vi "Log Data.vi"(8 "error in (no error)":errorcluster, 11 "Historian Logger in":refnum<class "Historian Logger.lvclass">) -> (0 "error out":errorcluster, 3 "Historian Logger out":refnum<class "Historian Logger.lvclass">)   [LabVIEW 2020, in "VolatusHistorian.lvlib" / "Historian Logger.lvclass"]
uses:
  Historian Logger.lvclass
  Historian Logger.lvclass/Historian Logger.ctl
  lv-vecto/Vecto/Group DBL/Group DBL.lvclass
  Volatus/MessageQ/MessageQ.lvclass/MessageQ.ctl
  Volatus/MessageQ/Send.vi
  lv-vecto/Vecto/Group/Group.lvclass
  VolatusData/VolatusData.lvlib
  VolatusErrorUtilities/MultiErrors/MultiErrors.lvclass
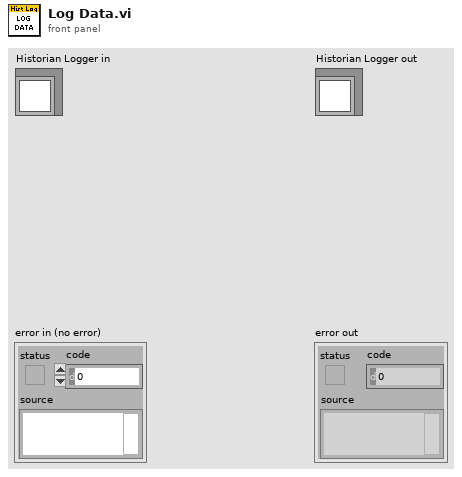
[diagram p1: front panel]
types:
  T1 = typedef "VolatusHistorian.lvlib/Historian Logger.lvclass/Group Info.ctl" = cluster{"Buffer":refnum<class "Group Buffer DBL.lvclass">, "Logger":refnum<class "MessageQ.lvclass">, "Group":refnum<class "Group.lvclass">, "Last Timestamp":dbl, "State":T2}
  T2 = typedef "VolatusData.lvlib/Logger State.ctl" = enum16{"Unknown", "Idle", "Preparing", "Ready", "Logging", "Stopping"}
  T3 = typedef "VectoConfig.lvlib/Group Data Type.ctl" = enum16{"Double", "String", "Bool"}
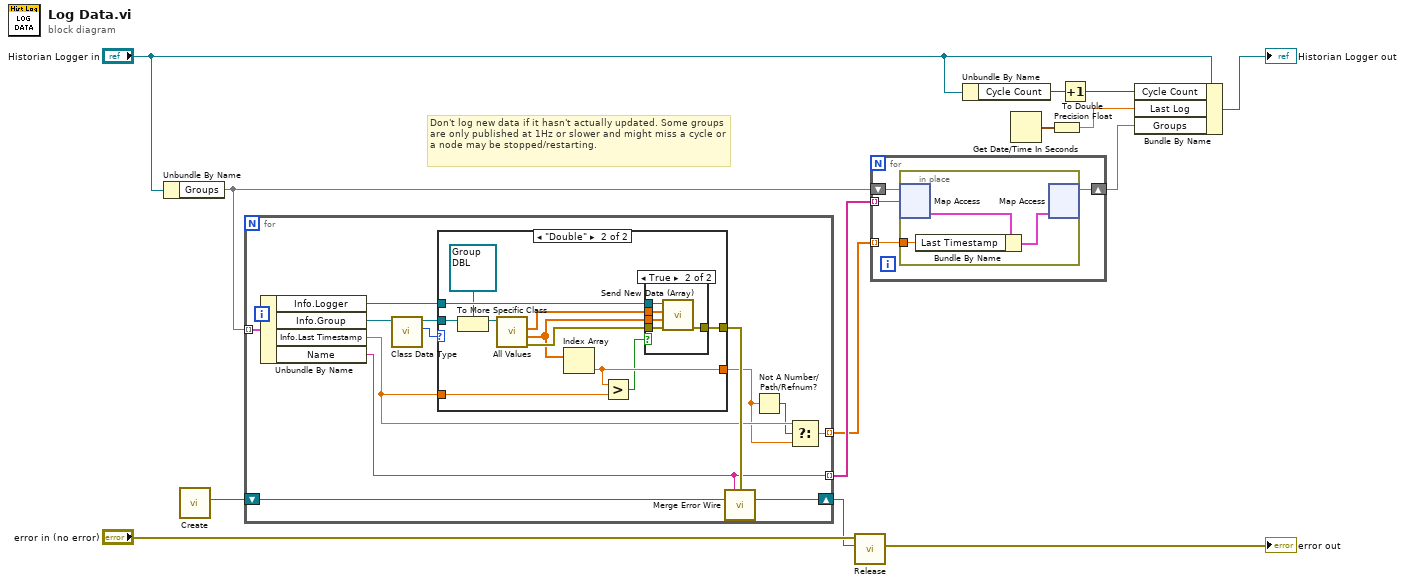
[diagram p0: block diagram]
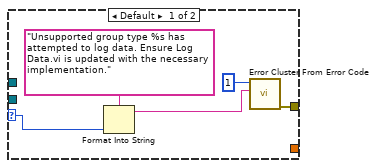
[diagram p2: hidden frame]
diagram:
  # "Don't log new data if it hasn't actually updated. Some groups are only published at 1Hz or slower and might miss a cycle or a node may be stopped/restarting."
  n1 = Unbundle By Name("Historian Logger in") -> ("Groups"=w4:map{string, T1})
  n2 = call "Create.vi"() -> ("MultiErrors out"=w14:refnum<class "MultiErrors.lvclass">)  [unwired: 11 in]
  n3 = for {
    tunnel: w4 -> [w27] mode=indexing
    shift-right: [w23] -> w11
    shift-left: w14 -> [w24]
    tunnel: [w15] -> w2 mode=indexing
    tunnel: [w22] -> w3 mode=indexing
    n4 = Unbundle By Name(w27) -> ("Info.Logger"=w26:refnum<class "MessageQ.lvclass">, "Info.Group"=w21:refnum<class "Group.lvclass">, "Info.Last Timestamp"=w18:dbl, "Name"=w22:string)
    n5 = call "Class Data Type.vi"("Group in"=w21) -> ("Class Data Type"=w20:T3, "Group out"=w19:refnum<class "Group.lvclass">)  [unwired: 8 in, 1 out]
    n6 = case shown="\"Double\"" w20 {
      selector: w20 -> [w29 _]
      tunnel: w26 -> [_ w43]
      tunnel: [w32 w40] -> w25
      tunnel: [_ w38] -> w16
      tunnel: w18 -> [_ w37]
      tunnel: w19 -> [_ w35]
      frame Default {
        n7 = Format Into String(format string="Unsupported group type %s has attempted to log data. Ensure Log Data.vi is updated with the necessary implementation.", w29) -> (resulting string=w28:string)  [unwired: 2 in, 1 out]
        n8 = call <vilib>:"Error Cluster From Error Code.vi"("error message (\"\")"=w28, "error code (0)"=1) -> ("error out"=w32:errorcluster)  [unwired: 7 in]
      }
      frame "Double" {
        n9 = To More Specific Class(target class=refnum<class "Group DBL.lvclass"> refnum ("Group in"), reference=w35) -> (specific class reference=w33:refnum<class "Group DBL.lvclass">)  [unwired: 1 in, 1 out]
        n10 = call "All Values.vi"("Group in"=w33) -> ("error out"=w41:errorcluster, "Timestamp"=w39:dbl[], "Scaled"=w42:dbl[])  [unwired: 6 in, 2 out]
        n11 = Index Array(array=w39) -> (element=w38:dbl)  [unwired: 1 in]
        n12 = Greater?(x=w38, y=w37) -> (0:w36:bool)
        n13 = case shown="True" w36 {
          tunnel: w43 -> [_ w49]
          tunnel: w42 -> [_ w48]
          tunnel: w41 -> [w44 w47]
          tunnel: [w44 w46] -> w40
          tunnel: w39 -> [_ w45]
          frame False {
          }
          frame True {
            n14 = call "Send New Data (Array).vi"("error in (no error)"=w47, "Timestamps (Now)"=w45, "Data"=w48, "MessageQ"=w49) -> ("error out"=w46:errorcluster)  [unwired: 7 in]
          }
        }
      }
    }
    n15 = call "Merge Error Wire.vi"("Local Context (None)"=w22, "error in (no error)"=w25, "MultiErrors in"=w24) -> ("MultiErrors out"=w23:refnum<class "MultiErrors.lvclass">)  [unwired: 12 in]
    n16 = Not A Number/Path/Refnum?(number/path/refnum=w16) -> (NaN/Path/Refnum?=w17:bool)
    n17 = Select(t=w18, s=w17, f=w16) -> (s? t:f=w15:dbl)
  }
  n18 = call "Release.vi"("MultiErrors in"=w11, "Upstream Error (None)"="error in (no error)") -> ("error out"=→"error out":errorcluster)  [unwired: 9 in]
  n19 = for {
    shift-right: [w50] -> w1
    shift-left: w4 -> [w53]
    tunnel: w3 -> [w52] mode=indexing
    tunnel: w2 -> [w51] mode=indexing
    n20 = in-place {
      in-place-border: w51 -> [w55]
      n21 = in-place-map #1(w53, w52) -> (w56:T1)  [unwired: 1 in, 1 out]
      n22 = Bundle By Name(cluster=w56, "Last Timestamp"=w55) -> (w54:T1)
      n23 = in-place-map #1(w54) -> (w50:map{string, T1})  [unwired: 1 in, 2 out]
    }
  }
  n24 = Unbundle By Name("Historian Logger in") -> ("Cycle Count"=w7:i32)
  n25 = Get Date/Time In Seconds() -> (seconds since 1Jan1904=w10:timestamp)
  n26 = To Double Precision Float(number=w10) -> (double precision float=w8:dbl)
  n27 = Increment(x=w7) -> (x+1=w6:i32)
  n28 = Bundle By Name(cluster="Historian Logger in", "Cycle Count"=w6, "Last Log"=w8, "Groups"=w1) -> (→"Historian Logger out":refnum<class "Historian Logger.lvclass">)
